vi "LWESP301_Open.vi"(6 "Instrument Key IN":string) -> (0 "error out":errorcluster, 1 "Error":i32, 2 "Instrument Key OUT":string, 3 "ESP301 Reference":refnum<k24>)   [LabVIEW 2010]
uses:
  C:/PVCS/IHM_Visual_Studio_NET/MotionControl/ESP301/Distribution/LabView/Source code/Dll/Newport.ESP301.CommandInterface.DLL
  Dll/Newport.ESP301.CommandInterface.DLL
panel:
  out "InstrumentKeys":string[](array[string])
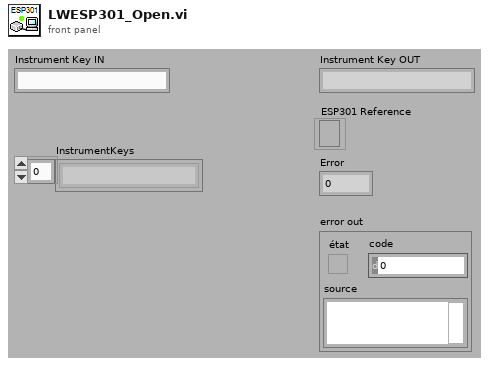
[diagram p1: front panel]
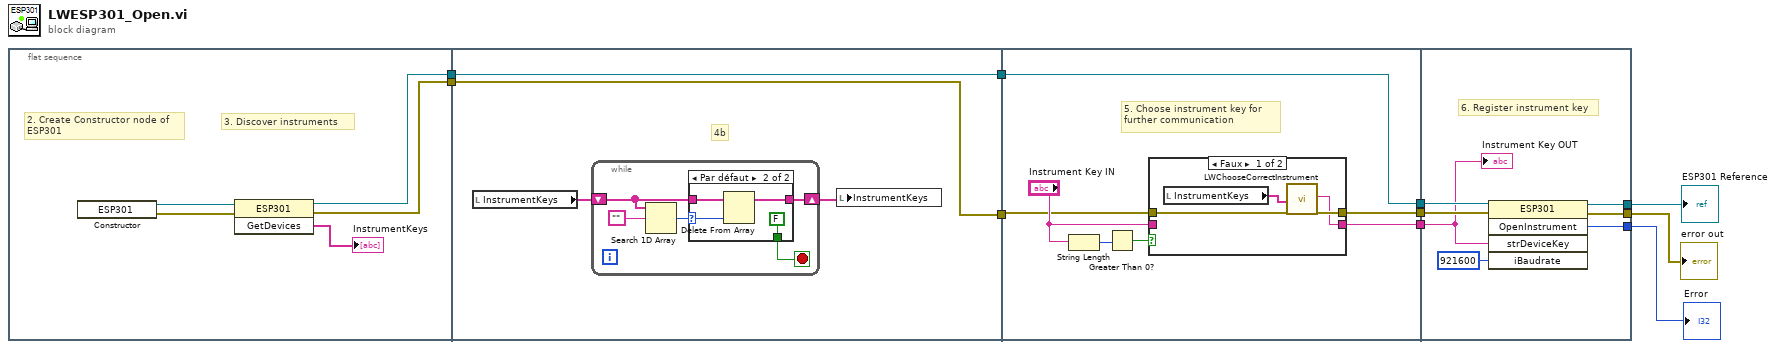
[diagram p0: block diagram]
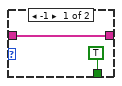
[diagram p2: hidden frame]
diagram:
  n1 = flat-sequence {
    tunnel: [w13] -> w5
    tunnel: [w12] -> w4
    tunnel: w4 -> [w17]
    tunnel: w5 -> [w16]
    tunnel: [w17] -> w8
    tunnel: [w16] -> w7
    tunnel: [w33] -> w10
    tunnel: [w32] -> w9
    tunnel: w8 -> [w34]
    tunnel: w7 -> [w33]
    tunnel: [w31] -> w6
    tunnel: w10 -> [w50]
    tunnel: w9 -> [w49]
    tunnel: w6 -> [w48]
    tunnel: [w46] -> w3
    tunnel: [w45] -> w2
    tunnel: [w44] -> w1
    frame #0 {
      # "3. Discover instruments"
      # "2. Create Constructor node of \nESP301"
      n2 = constructor class="ESP301"() -> (reference out=w15:refnum<k24>, error out=w14:errorcluster)  [unwired: 3 in, 1 out]
      n3 = invoke class="ESP301" method="GetDevices"(reference=w15, error in=w14) -> (reference out=w13:refnum<k24>, error out=w12:errorcluster, "GetDevices"=→"InstrumentKeys":string[])  [unwired: 1 in]
    }
    frame #1 {
      # "4b"
      n4 = local read "InstrumentKeys"() -> (w18:string[])
      n5 = while {
        shift-right: [w24] -> w19
        shift-left: w18 -> [w23]
        stop <- w21 stop-if-true
        n6 = Search 1D Array(1D array=w23, element="") -> (index of element=w22:i32)  [unwired: 1 in]
        n7 = case shown="Par défaut" w22 {
          selector: w22 -> [_ w28]
          tunnel: w23 -> [w26 w30]
          tunnel: [w26 w29] -> w24
          tunnel: [TRUE FALSE] -> w21
          frame -1 {
          }
          frame Default {
            n8 = Delete From Array(array=w30, index=w28) -> (array with subset deleted=w29:string[])  [unwired: 1 in, 1 out]
          }
        }
      }
      n9 = local write "InstrumentKeys"(w19) -> ()
    }
    frame #2 {
      # "5. Choose instrument key for \nfurther communication"
      n10 = String Length(string="Instrument Key IN") -> (length=w35:i32)
      n11 = Greater Than 0?(x=w35) -> (x > 0?=w36:bool)
      n12 = case shown="Faux" w36 {
        tunnel: w34 -> [w41 w43]
        tunnel: [w39 w43] -> w32
        tunnel: [w38 w42] -> w31
        tunnel: "Instrument Key IN" -> [_ w42]
        frame False {
          n13 = local read "InstrumentKeys"() -> (w40:string[])
          n14 = call "LWChooseCorrectInstrument.vi"("Instrument Keys"=w40, "error in (no error)"=w41) -> ("selected instrument key"=w38:string, "error out"=w39:errorcluster)  [unwired: 16 in]
        }
        frame True {
        }
      }
    }
    frame #3 {
      # "6. Register instrument key"
      n15 = invoke class="ESP301" method="OpenInstrument"(reference=w50, error in=w49, "strDeviceKey"=w48, "iBaudrate"=921600) -> (reference out=w46:refnum<k24>, error out=w45:errorcluster, "OpenInstrument"=w44:i32)  [unwired: 1 in, 2 out]
      "Instrument Key OUT" <- w48
    }
  }
  "error out" <- w2
  "ESP301 Reference" <- w3
  "Error" <- w1
